vi "Config.vi"(8 "Error In":errorcluster) -> (0 "Error Out":errorcluster)   [LabVIEW 2019, in "Full User Interface.lvlib"]
uses:
  Full User Interface.lvlib
  <vilib>/Test Bench Framework/Test Executive.lvlibp/TestEngine/TestEngine/TestEngine/Typedefs/Local Report Configuration.ctl
  <vilib>/Test Bench Framework/Test Executive.lvlibp/TestEngine/TestEngine/TestEngine/Report Format.ctl
  <vilib>/Test Bench Framework/Test Executive.lvlibp/TestEngine/TestEngine/TestEngine/Typedefs/Database Configuration.ctl
  <vilib>/Test Bench Framework/Test Executive.lvlibp/TestEngine/TestEngine/TestEngine/Typedefs/TestEngine Cofiguration.ctl
  <vilib>/Test Bench Framework/Test Executive.lvlibp/TestEngine/TestEngine/TestEngine/Test Engine.lvclass
panel:
  in  "Cancel":bool
  in  "OK":bool
  in  "Tab Control":enum32{"Local Report", "Database", "Execute"}(tab)
  in  "Local Report Configuration":T1
  in  "Database Configuration":T3
  in  "Execute":T4
  # "*不合格时结束测试"
  # "*运行的时候忽略断点"
  # "*过滤测试项目，只显示有测试结果的测试项"
  # "*自动错误处理，测试项报错\n  时不显示弹窗"
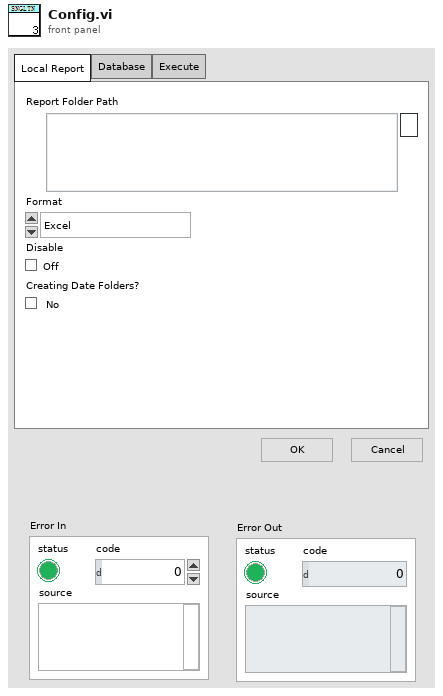
[diagram p1: front panel]
types:
  T1 = typedef "Test Executive.lvlibp/Test Engine.lvlib/Test Engine.lvclass/Local Report Configuration.ctl" = cluster{"Report Folder Path":path, "Format":T2, "Disable":bool, "Build Date Folder?":bool, "Execl Template Path":path}
  T2 = typedef "Test Executive.lvlibp/Test Engine.lvlib/Test Engine.lvclass/Report Format.ctl" = enum16{"Excel", "CSV(Tab)", "CSV(,)", "CSV(;)", "TEXT", "HTML"}
  T3 = typedef "Test Executive.lvlibp/Test Engine.lvlib/Test Engine.lvclass/Database Configuration.ctl" = cluster{"Connection String Expression":string, "Microsoft Data Link File":path, "Connection Type":enum16{"Use Connection String Expression", "Use Microsoft Data Link File"}, "Enable":bool}
  T4 = cluster{"Automatically handle TestVI error":cluster{"Enable":bool, "Handle":enum16{"Termination test", "Ignore error"}}, "Break on Failure":bool, "Ignore breakpoint":bool, "Filter Result":bool}
  T5 = enum32{"Invalid", "Standard", "Closed", "Hidden", "Minimized", "Maximized"}
  T6 = enum32{"invalid app kind", "Development System", "Run Time System", "Student Edition", "Embedded LabVIEW", "Evaluation", "Custom"}
  T7 = typedef "Test Executive.lvlibp/Test Engine.lvlib/Test Engine.lvclass/TestEngine Cofiguration.ctl" = cluster{"Break on Failure":bool, "Automatically handle TestVI error":cluster{"Enable":bool, "Handle":enum16{"Termination test", "Ignore error"}}, "Local Report Configuration":T1, "Database Configuration":T3, "Ignore breakpoint":bool, "Filter Result":bool}
  T8 = cluster{"Core":cluster{"Current VI Reference":refnum<vi>, "Close Panel on Exit?":bool}, "TestEngine Cofiguration":T7, "handle error":refnum<vi>, "Break on Failure":refnum<vi>, "Ignore breakpoint":refnum<vi>, "Filter Result":refnum<vi>, "Database Configuration":refnum<vi>, "Local Report Configuration":refnum<vi>, "Tab Control":refnum<vi>, "Execl Template Path":refnum<vi>}
  T9 = cluster{"Current VI Reference":refnum<vi>, "Close Panel on Exit?":bool}
  T10 = cluster{"Enable":bool, "Handle":enum16{"Termination test", "Ignore error"}}
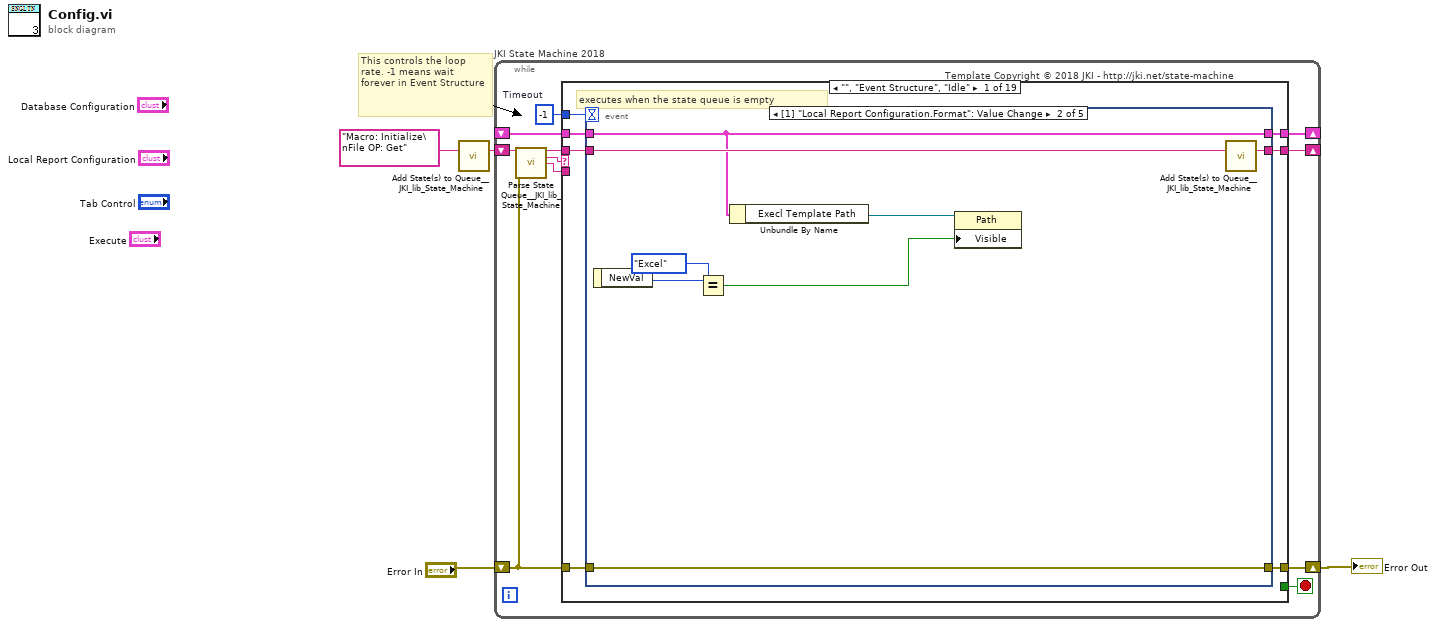
[diagram p0: block diagram]
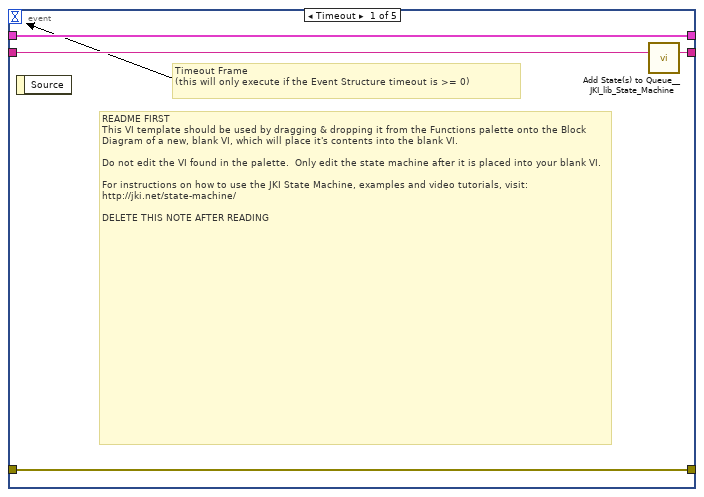
[diagram p2: hidden frame]
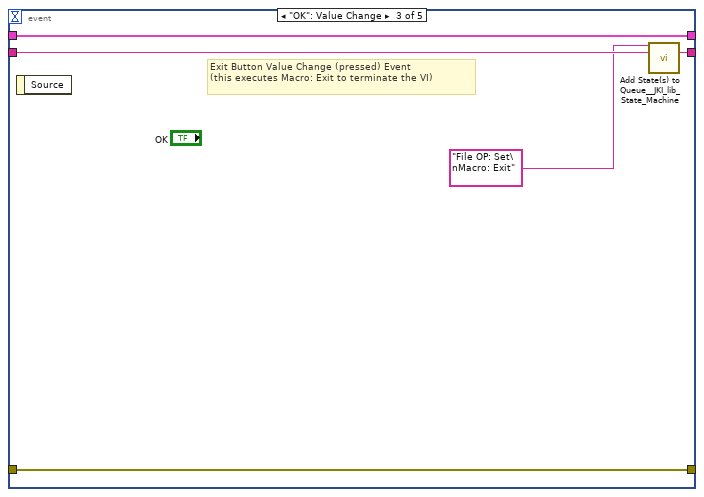
[diagram p3: hidden frame]
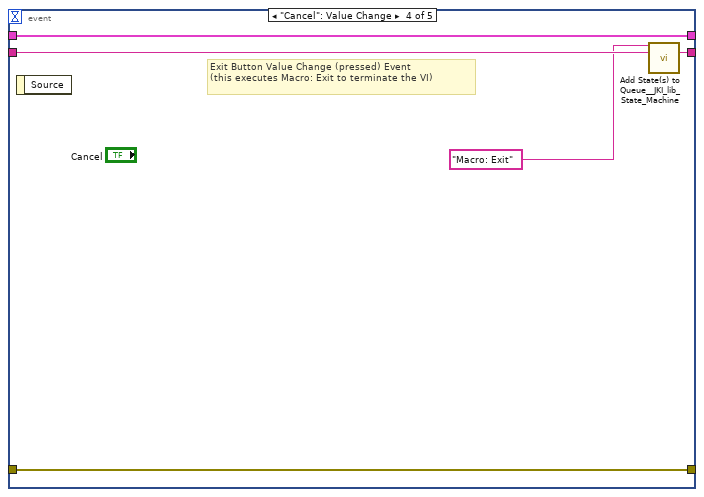
[diagram p4: hidden frame]
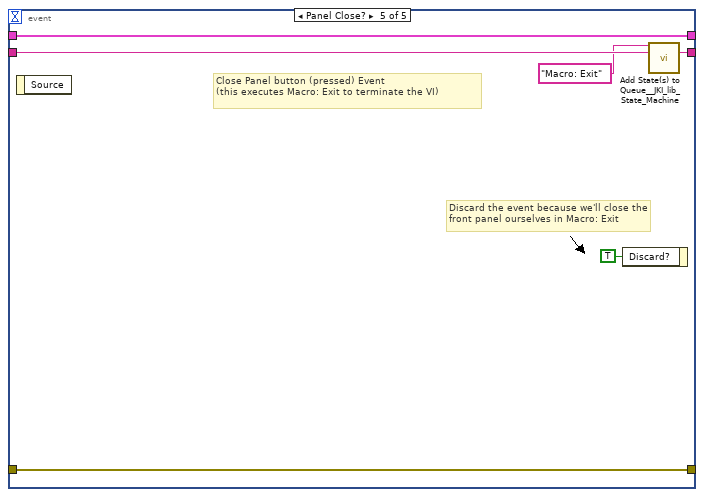
[diagram p5: hidden frame]
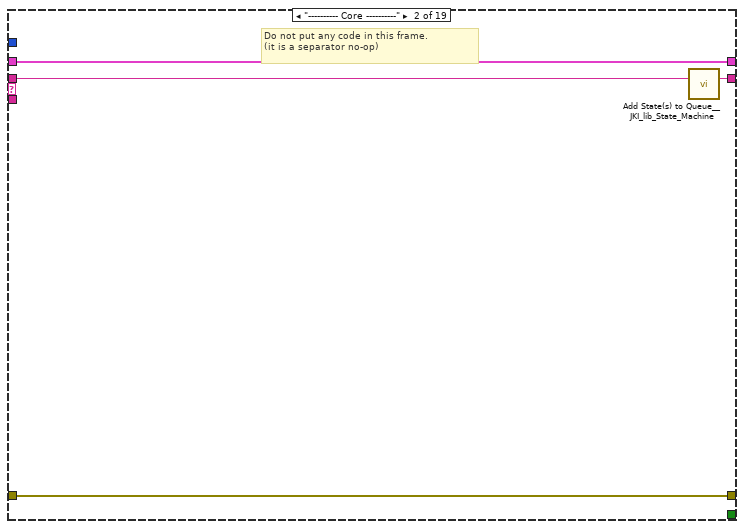
[diagram p6: hidden frame]
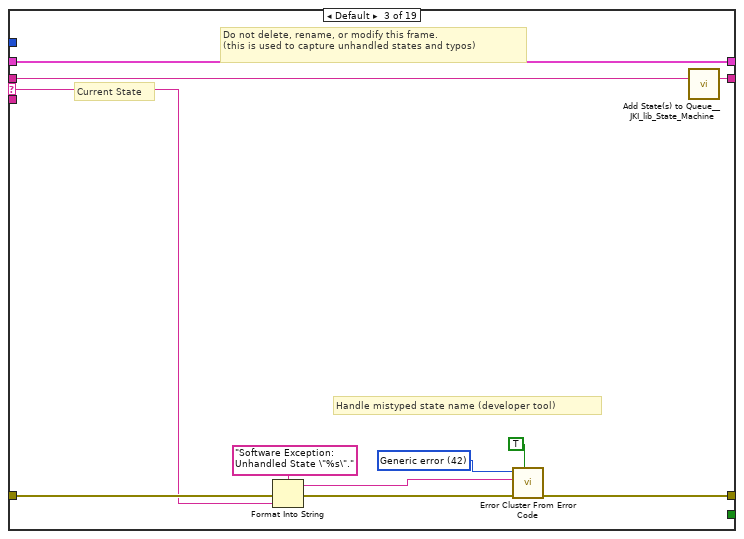
[diagram p7: hidden frame]
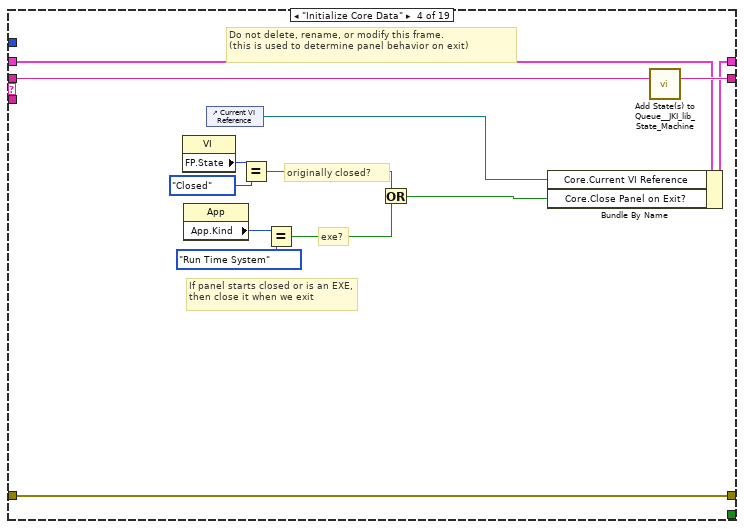
[diagram p8: hidden frame]
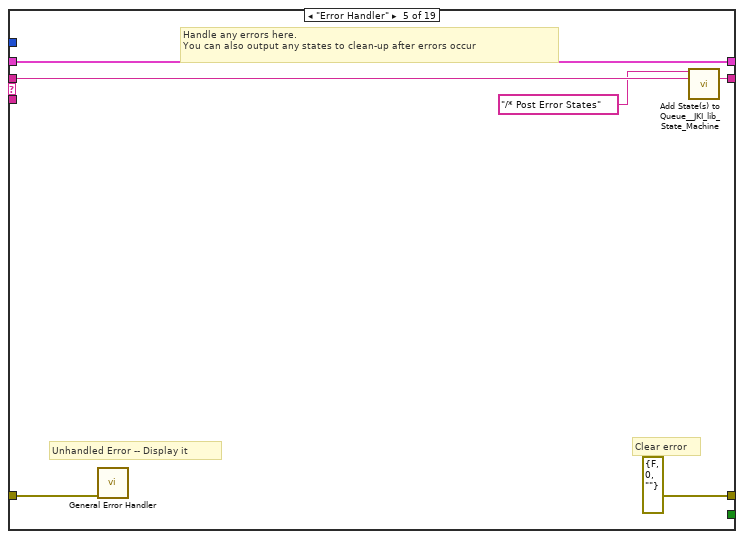
[diagram p9: hidden frame]
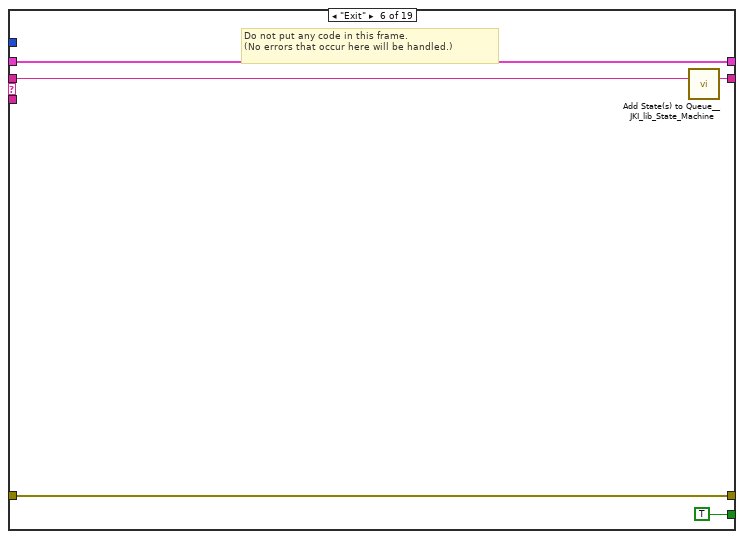
[diagram p10: hidden frame]
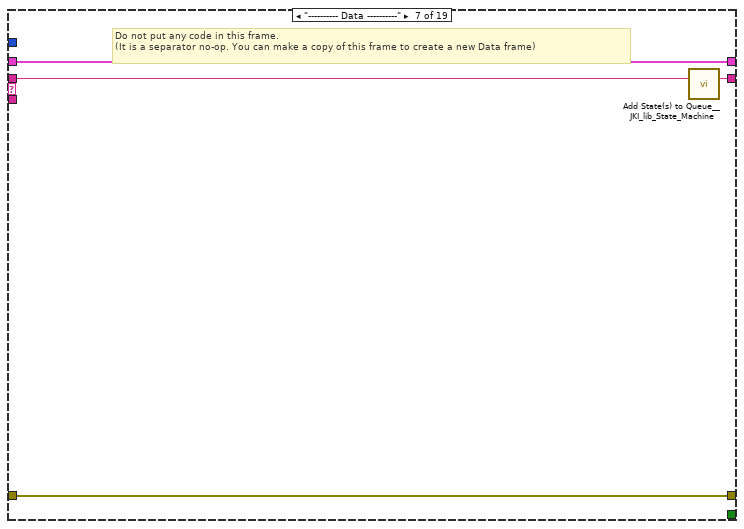
[diagram p11: hidden frame]
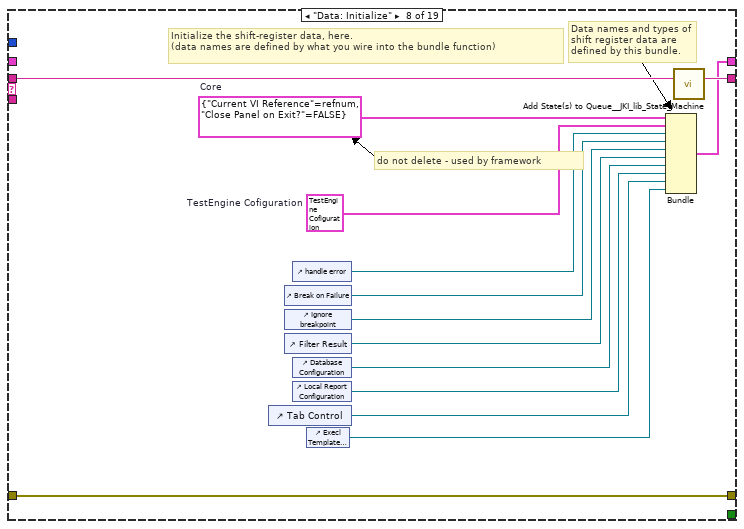
[diagram p12: hidden frame]
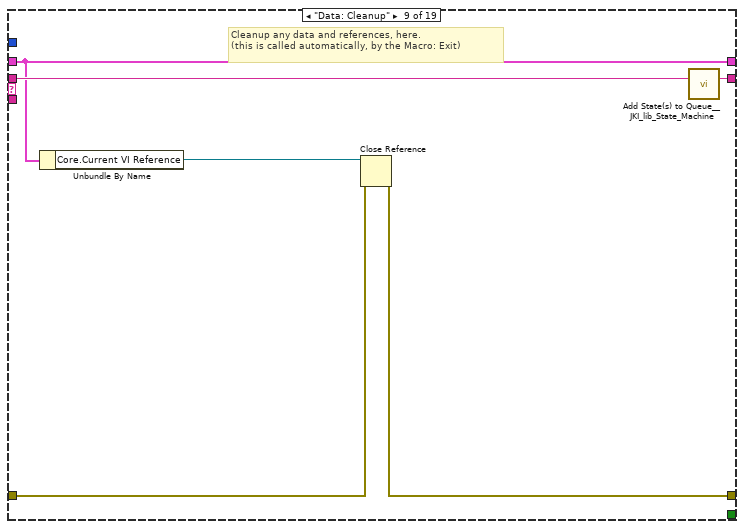
[diagram p13: hidden frame]
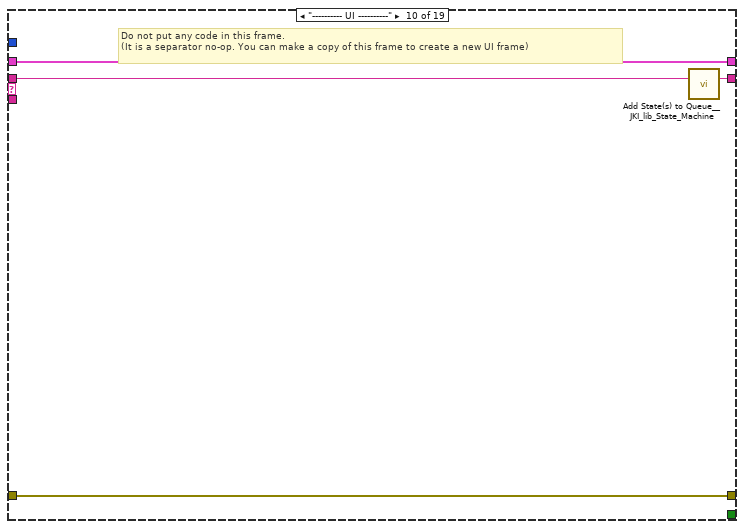
[diagram p14: hidden frame]
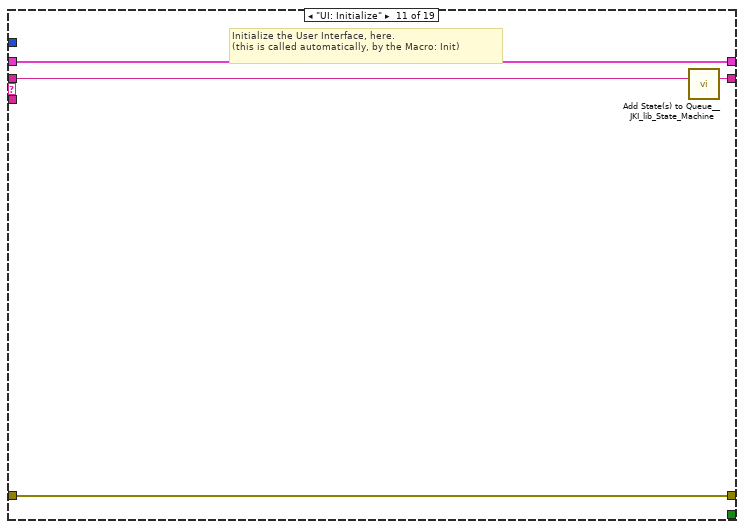
[diagram p15: hidden frame]
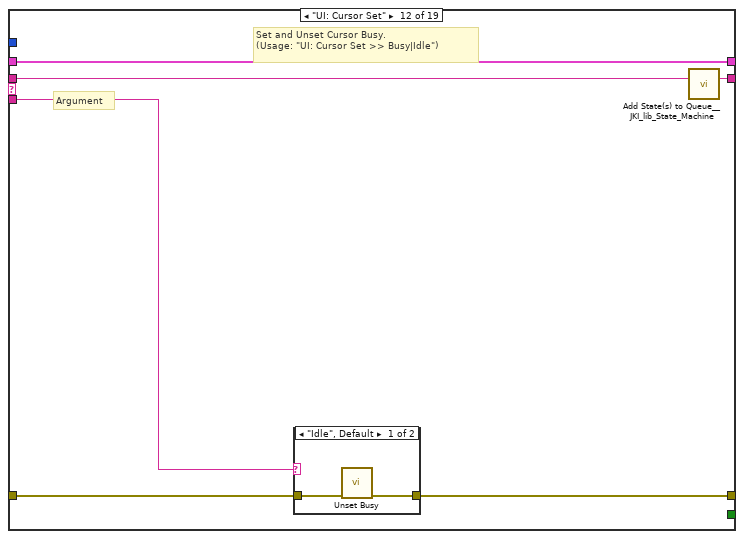
[diagram p16: hidden frame]
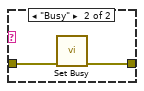
[diagram p17: hidden frame]
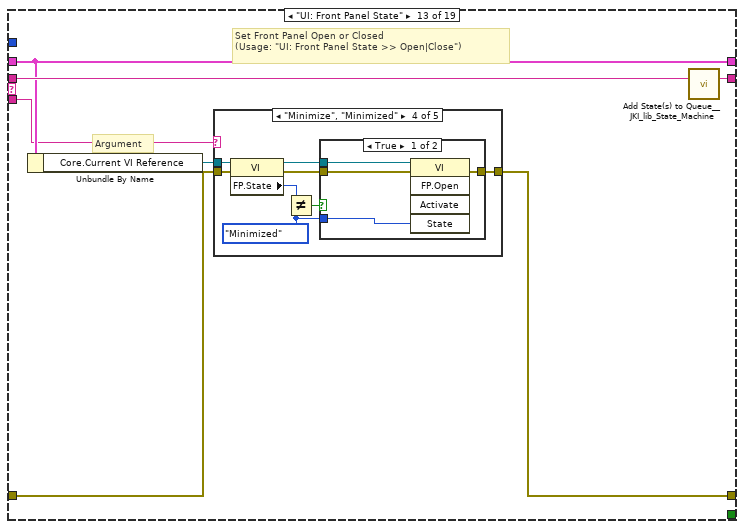
[diagram p18: hidden frame]
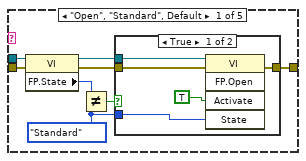
[diagram p19: hidden frame]
diagram:
  # "This controls the loop rate. -1 means wait forever in Event Structure"
  n1 = call <vilib>:"Add State(s) to Queue__JKI_lib_State_Machine.vi"("State(s) in (\"\")"="Macro: Initialize\nFile OP: Get") -> ("States Out"=w4:string)  [unwired: 14 in]
  n2 = while "JKI State Machine 2018" {
    shift-right: [w8] -> _
    shift-left: _ -> [w7]
    shift-right: [w11] -> w1
    shift-left: "Error In" -> [w5]
    shift-right: [w10] -> _
    shift-left: w4 -> [w12]
    stop <- w9 stop-if-true
    w6 = -1  # Timeout
    # "Template Copyright © 2018 JKI - http://jki.net/state-machine"
    n3 = call <vilib>:"Parse State Queue__JKI_lib_State_Machine.vi"("State Queue"=w12, "Error In (no error)"=w5) -> ("Remaining States"=w14:string, "Current State"=w15:string, "Arguments"=w13:string)  [unwired: 11 in]
    n4 = case shown="\"\", \"Event Structure\", \"Idle\"" w15 {
      selector: w15 -> [_ _ w55 _ _ _ _ _ _ _ _ _ _ _ _ _ _ _ _]
      tunnel: w14 -> [w22 w54 w59 w78 w84 w89 w93 w107 w113 w117 w121 w127 w138 w207 w212 w222 w226 w249 w269]
      tunnel: w13 -> [_ _ _ _ _ _ _ _ _ _ _ w122 w132 _ _ _ _ _ _]
      tunnel: w7 -> [w20 w51 w57 w71 w81 w87 w90 _ w108 w114 w119 w125 w134 w204 w209 w219 w223 w246 w260]
      tunnel: [w19 w52 w61 w75 errorcluster {"status"=FALSE, "code"=0, "source"=""} ("error out") w86 w91 w104 w109 w115 w118 w123 w135 w205 w210 w220 w224 w245 w252] -> w11
      tunnel: w5 -> [w18 w52 w60 w75 w80 w86 w91 w104 w110 w115 w118 w124 w136 w205 w210 w220 w224 w247 w267]
      tunnel: [w21 w53 w58 w77 w83 w88 w92 w106 w112 w116 w120 w126 w137 w206 w211 w221 w225 w248 w268] -> w10
      tunnel: [_ _ _ _ _ TRUE _ _ _ _ _ _ _ _ _ _ _ _ _] -> w9
      tunnel: [w17 w51 w57 w76 w81 w87 w90 w105 w108 w114 w119 w125 w134 w204 w209 w219 w223 w246 w260] -> w8
      tunnel: w6 -> [w16 _ _ _ _ _ _ _ _ _ _ _ _ _ _ _ _ _ _]
      frame "", "Event Structure", "Idle" {
        # "executes when the state queue is empty"
        n5 = event shown="[1] \"Local Report Configuration.Format\": Value Change" {
          selector: _ -> [_ _ _ _ _]
          dyn-events: _ -> [_ _ _ _ _]
          timeout: w16 -> [_ _ _ _ _]
          tunnel: w22 -> [w26 w34 w39 w44 w50]
          tunnel: [w25 w33 w38 w43 w49] -> w21
          tunnel: w20 -> [w23 w29 w36 w41 w47]
          tunnel: [w24 w32 w37 w42 w48] -> w19
          tunnel: w18 -> [w24 w32 w37 w42 w48]
          tunnel: [w23 w29 w36 w41 w47] -> w17
          event Timeout {
            # "README FIRST\nThis VI template should be used by dragging & dropping it from the Functions palette onto the Block Diagram of a new, blank VI, which will place it's contents into the blank VI.\n\nDo not edit the VI found in the palette.  Only edit the state machine after it is placed into your blank VI.\n\nFor instructions on how to use the JKI State Machine, examples and video tutorials, visit:\nhttp://jki.net/state-machine/\n\nDELETE THIS NOTE AFTER READING"
            # "Timeout Frame\n(this will only execute if the Event Structure timeout is >= 0)"
            n6 = event-data() -> ()  [unwired: 1 in, 1 out]
            n7 = call <vilib>:"Add State(s) to Queue__JKI_lib_State_Machine.vi"("State(s) in (\"\")"=w26) -> ("States Out"=w25:string)  [unwired: 14 in]
          }
          event Value Change {
            n8 = event-data() -> ("NewVal"=w31:T2)  [unwired: 1 in]
            n9 = Equal?(x=w31, y=Report_Format."Excel") -> (x = y?=w27:bool)
            n10 = Unbundle By Name(w29) -> ("Execl Template Path"=w28:refnum<vi>)
            n11 = property class="Path"(reference=w28, "Visible"=w27) -> ()  [unwired: 1 in, 2 out]
            n12 = call <vilib>:"Add State(s) to Queue__JKI_lib_State_Machine.vi"("State(s) in (\"\")"=w34) -> ("States Out"=w33:string)  [unwired: 14 in]
          }
          event "OK": Value Change {
            # "Exit Button Value Change (pressed) Event\n(this executes Macro: Exit to terminate the VI)"
            n13 = event-data() -> ()  [unwired: 1 in, 1 out]
            n14 = call <vilib>:"Add State(s) to Queue__JKI_lib_State_Machine.vi"("State(s) in Front (\"\")"="File OP: Set\nMacro: Exit", "State(s) in (\"\")"=w39) -> ("States Out"=w38:string)  [unwired: 13 in]
          }
          event "Cancel": Value Change {
            # "Exit Button Value Change (pressed) Event\n(this executes Macro: Exit to terminate the VI)"
            n15 = event-data() -> ()  [unwired: 1 in, 1 out]
            n16 = call <vilib>:"Add State(s) to Queue__JKI_lib_State_Machine.vi"("State(s) in Front (\"\")"="Macro: Exit", "State(s) in (\"\")"=w44) -> ("States Out"=w43:string)  [unwired: 13 in]
          }
          event Panel Close? {
            # "Discard the event because we'll close the front panel ourselves in Macro: Exit"
            # "Close Panel button (pressed) Event\n(this executes Macro: Exit to terminate the VI)"
            n17 = event-data() -> ()  [unwired: 1 in, 1 out]
            n18 = event-data("Discard?"=TRUE) -> ()  [unwired: 1 in, 1 out]
            n19 = call <vilib>:"Add State(s) to Queue__JKI_lib_State_Machine.vi"("State(s) in Front (\"\")"="Macro: Exit", "State(s) in (\"\")"=w50) -> ("States Out"=w49:string)  [unwired: 13 in]
          }
        }
      }
      frame "---------- Core ----------" {
        # "Do not put any code in this frame.\n(it is a separator no-op)"
        n20 = call <vilib>:"Add State(s) to Queue__JKI_lib_State_Machine.vi"("State(s) in (\"\")"=w54) -> ("States Out"=w53:string)  [unwired: 14 in]
      }
      frame Default {
        w64 = 42 items=["No error", "Argument error", "Memory is full", "Out of zone", "End of file", "File already open", "Generic file I/O error", "File not found", "File permission error", "Disk is full", "Duplicate path", "Too many files open", "System feature not enabled", "Resource file not found", "Cannot add resource", "Resource not found", "Image not found", "Image memory error", "Pen does not exist", "Config type invalid", "Config token not found", "Config parse error", "Config memory error", "Bad external code format", "Bad external code offset", "External code not present", "Null window", "Destroy window error", "Null menu", "Print aborted", "Bad print record", "Print driver error", "Windows error during printing", "Memory error during printing", "Print dialog error", "Generic print error", "Invalid device refnum", "Device not found", "Device parameter error", "Device unit error", "Cannot open device", "Device call aborted", "Generic error", "Cancelled by user", "Object ID too low", "Object ID too high", "Object not in heap", "Unknown heap", "Unknown object (invalid DefProc)", "Unknown object (DefProc not in table)", "Message out of range", "Invalid (null) method", "Unknown message", "Manager call not supported", "Bad address", "Network operation in progress", "Network operation timed out", "Connection is busy", "Network attribute not supported", "Network error", "Address in use", "System out of memory", "Connection aborted", "Connection refused", "Not connected", "Already connected", "Connection closed", "Initialization error (interapplication manager)", "Bad occurrence", "Wait on unbound occurrence handler", "Occurrence queue overflow", "Datalog type conflict", "Unused", "Unrecognized type (interapplication manager)", "Memory corrupt", "Failed to make temporary DLL", "Old CIN version", "Drag socket not found", "Failed to load drop-object", "Failed to register OLE object", "Failed to release OLE object", "Format specifier type mismatch", "Unknown format specifier", "Too few format specifiers", "Too many format specifiers", "Scan failed", "Newer CIN version", "Error converting to variant", "Runtime menu error", "Password tampered", "Variant attribute not found", "Incompatible variant data type", "Event data is not available", "Event Store is not present", "Occurrence is not found", "Event Queue is not created", "Event info is not available", "Refnum passed is NULL", "Error retrieving Class GUID", "Error retrieving CoClass GUID", "Error retrieving TypeLib GUID.", "Bad built application magic bytes.", "Specific driver is different from the specific driver associated with the Logical Name.", "There is no session opened to the class driver.", "Max Error", "MAX - Error with config objects", "MAX - Error loading configuration", "MAX - Group not supported"]
        # "Current State"
        # "Do not delete, rename, or modify this frame.\n(this is used to capture unhandled states and typos)"
        # "Handle mistyped state name (developer tool)"
        n21 = Format Into String(format string="Software Exception: Unhandled State \"%s\"." ("message"), error in=w60, w55) -> (resulting string=w63:string, error out=w62:errorcluster)  [unwired: 1 in]
        n22 = call <vilib>:"Error Cluster From Error Code.vi"("show call chain? (False)"=TRUE, "error in (no error)"=w62, "error message (\"\")"=w63, "error code (0)"=w64) -> ("error out"=w61:errorcluster)  [unwired: 5 in]
        n23 = call <vilib>:"Add State(s) to Queue__JKI_lib_State_Machine.vi"("State(s) in (\"\")"=w59) -> ("States Out"=w58:string)  [unwired: 14 in]
      }
      frame "Initialize Core Data" {
        # "Do not delete, rename, or modify this frame.\n(this is used to determine panel behavior on exit)"
        # "originally closed?"
        # "exe?"
        # "If panel starts closed or is an EXE, then close it when we exit"
        n24 = property class="VI"() -> ("FP.State"=w68:T5)  [unwired: 2 in, 2 out]
        n25 = property class="App"() -> ("App.Kind"=w74:T6)  [unwired: 2 in, 2 out]
        n26 = control-ref of="Current VI Reference"() -> (w69:refnum<vi>)
        n27 = Equal?(x=w68, y=T5."Closed" ("Front Panel Window:State")) -> (x = y?=w66:bool)
        n28 = Equal?(x=w74, y=T6."Run Time System" ("Application:Kind")) -> (x = y?=w72:bool)
        n29 = Or(x=w66, y=w72) -> (x .or. y?=w70:bool)
        n30 = Bundle By Name(cluster=w71, "Core.Current VI Reference"=w69, "Core.Close Panel on Exit?"=w70) -> (w76:T8)
        n31 = call <vilib>:"Add State(s) to Queue__JKI_lib_State_Machine.vi"("State(s) in (\"\")"=w78) -> ("States Out"=w77:string)  [unwired: 14 in]
      }
      frame "Error Handler" {
        # "Unhandled Error -- Display it"
        # "Handle any errors here.\nYou can also output any states to clean-up after errors occur"
        # "Clear error"
        n32 = call <vilib>:"General Error Handler.vi"("error in (no error)"=w80) -> ()  [unwired: 10 in, 5 out]
        n33 = call <vilib>:"Add State(s) to Queue__JKI_lib_State_Machine.vi"("State(s) in Front (\"\")"="/* Post Error States", "State(s) in (\"\")"=w84) -> ("States Out"=w83:string)  [unwired: 13 in]
      }
      frame "Exit" {
        # "Do not put any code in this frame.\n(No errors that occur here will be handled.)"
        n34 = call <vilib>:"Add State(s) to Queue__JKI_lib_State_Machine.vi"("State(s) in (\"\")"=w89) -> ("States Out"=w88:string)  [unwired: 14 in]
      }
      frame "---------- Data ----------" {
        # "Do not put any code in this frame.\n(It is a separator no-op. You can make a copy of this frame to create a new Data frame)"
        n35 = call <vilib>:"Add State(s) to Queue__JKI_lib_State_Machine.vi"("State(s) in (\"\")"=w93) -> ("States Out"=w92:string)  [unwired: 14 in]
      }
      frame "Data: Initialize" {
        w102 = T7 {"Break on Failure"=FALSE, "Automatically handle TestVI error"={"Enable"=FALSE, "Handle"=enum."Termination test"}, "Local Report Configuration"={"Report Folder Path"=path "", "Format"=enum."Excel", "Disable"=FALSE, "Build Date Folder?"=FALSE, "Execl Template Path"=path ""}, "Database Configuration"={"Connection String Expression"="", "Microsoft Data Link File"=path "", "Connection Type"=enum."Use Connection String Expression", "Enable"=FALSE}, "Ignore breakpoint"=FALSE, "Filter Result"=FALSE}  # TestEngine Cofiguration
        w103 = T9 {"Current VI Reference"=refnum, "Close Panel on Exit?"=FALSE}  # Core
        # "do not delete - used by framework"
        # "Data names and types of shift register data are defined by this bundle."
        # "Initialize the shift-register data, here.\n(data names are defined by what you wire into the bundle function)"
        n36 = control-ref of="Tab Control"() -> (w95:refnum<vi>)
        n37 = control-ref of="Break on Failure"() -> (w100:refnum<vi>)
        n38 = control-ref of="Ignore breakpoint"() -> (w99:refnum<vi>)
        n39 = control-ref of="Filter Result"() -> (w98:refnum<vi>)
        n40 = control-ref of="handle error"() -> (w101:refnum<vi>)
        n41 = control-ref of="Database Configuration"() -> (w97:refnum<vi>)
        n42 = control-ref of="Local Report Configuration"() -> (w96:refnum<vi>)
        n43 = control-ref of="Execl Template Path"() -> (w94:refnum<vi>)
        n44 = Bundle("Core"=w103, "TestEngine Cofiguration"=w102, "handle error"=w101, "Break on Failure"=w100, "Ignore breakpoint"=w99, "Filter Result"=w98, "Database Configuration"=w97, "Local Report Configuration"=w96, "Tab Control"=w95, "Execl Template Path"=w94) -> (w105:T8)  [unwired: 1 in]
        n45 = call <vilib>:"Add State(s) to Queue__JKI_lib_State_Machine.vi"("State(s) in (\"\")"=w107) -> ("States Out"=w106:string)  [unwired: 14 in]
      }
      frame "Data: Cleanup" {
        # "Cleanup any data and references, here.\n(this is called automatically, by the Macro: Exit)"
        n46 = Unbundle By Name(w108) -> ("Core.Current VI Reference"=w111:refnum<vi>)
        n47 = Close Reference(reference=w111, error in (no error)=w110) -> (error out=w109:errorcluster)
        n48 = call <vilib>:"Add State(s) to Queue__JKI_lib_State_Machine.vi"("State(s) in (\"\")"=w113) -> ("States Out"=w112:string)  [unwired: 14 in]
      }
      frame "---------- UI ----------" {
        # "Do not put any code in this frame.\n(It is a separator no-op. You can make a copy of this frame to create a new UI frame)"
        n49 = call <vilib>:"Add State(s) to Queue__JKI_lib_State_Machine.vi"("State(s) in (\"\")"=w117) -> ("States Out"=w116:string)  [unwired: 14 in]
      }
      frame "UI: Initialize" {
        # "Initialize the User Interface, here.\n(this is called automatically, by the Macro: Init)"
        n50 = call <vilib>:"Add State(s) to Queue__JKI_lib_State_Machine.vi"("State(s) in (\"\")"=w121) -> ("States Out"=w120:string)  [unwired: 14 in]
      }
      frame "UI: Cursor Set" {
        # "Argument"
        # "Set and Unset Cursor Busy.\n(Usage: \"UI: Cursor Set >> Busy|Idle\")"
        n51 = case shown="\"Idle\", Default" w122 {
          tunnel: w124 -> [w129 w131]
          tunnel: [w128 w130] -> w123
          frame "Idle", Default {
            n52 = call <vilib>:"Unset Busy.vi"("error in (no error)"=w129) -> ("error out"=w128:errorcluster)  [unwired: 10 in]
          }
          frame "Busy" {
            n53 = call <vilib>:"Set Busy.vi"("error in (no error)"=w131) -> ("error out"=w130:errorcluster)  [unwired: 9 in, 1 out]
          }
        }
        n54 = call <vilib>:"Add State(s) to Queue__JKI_lib_State_Machine.vi"("State(s) in (\"\")"=w127) -> ("States Out"=w126:string)  [unwired: 14 in]
      }
      frame "UI: Front Panel State" {
        # "Argument"
        # "Set Front Panel Open or Closed\n(Usage: \"UI: Front Panel State >> Open|Close\")"
        n55 = Unbundle By Name(w134) -> ("Core.Current VI Reference"=w133:refnum<vi>)
        n56 = case shown="\"Minimize\", \"Minimized\"" w132 {
          tunnel: w136 -> [w144 w159 w170 w183 w196]
          tunnel: [w146 w160 w172 w185 w198] -> w135
          tunnel: w133 -> [w145 w157 w171 w184 w197]
          frame "Open", "Standard", Default {
            w139 = T5."Standard" ("State")
            n57 = property class="VI"(reference=w145, error in=w144) -> (reference out=w142:refnum<vi>, error out=w143:errorcluster, "FP.State"=w141:T5)
            n58 = Not Equal?(x=w141, y=w139) -> (x != y?=w140:bool)
            n59 = case shown="True" w140 {
              tunnel: [w150 w152] -> w146
              tunnel: w143 -> [w149 w152]
              tunnel: w142 -> [w148 _]
              tunnel: w139 -> [w147 _]
              frame True {
                n60 = invoke class="VI" method="FP.Open"(reference=w148, error in=w149, "Activate"=TRUE, "State"=w147) -> (error out=w150:errorcluster)  [unwired: 1 in, 4 out]
              }
              frame False {
              }
            }
          }
          frame "Close", "Closed" {
            n61 = property class="VI"(reference=w157, error in=w159) -> (reference out=w156:refnum<vi>, error out=w158:errorcluster, "FP.State"=w154:T5)
            n62 = Not Equal?(x=w154, y=T5."Closed" ("Front Panel Window:State")) -> (x != y?=w153:bool)
            n63 = case shown="True" w153 {
              tunnel: [w161 w164] -> w160
              tunnel: w158 -> [w161 w163]
              tunnel: w156 -> [_ w162]
              frame False {
              }
              frame True {
                n64 = invoke class="VI" method="FP.Close"(reference=w162, error in=w163) -> (error out=w164:errorcluster)  [unwired: 1 in, 2 out]
              }
            }
          }
          frame "Hidden", "Hide" {
            w165 = T5."Hidden" ("State")
            n65 = property class="VI"(reference=w171, error in=w170) -> (reference out=w168:refnum<vi>, error out=w169:errorcluster, "FP.State"=w167:T5)
            n66 = Not Equal?(x=w167, y=w165) -> (x != y?=w166:bool)
            n67 = case shown="True" w166 {
              tunnel: [w176 w177] -> w172
              tunnel: w169 -> [w175 w177]
              tunnel: w168 -> [w174 _]
              tunnel: w165 -> [w173 _]
              frame True {
                n68 = invoke class="VI" method="FP.Open"(reference=w174, error in=w175, "State"=w173) -> (error out=w176:errorcluster)  [unwired: 2 in, 4 out]
              }
              frame False {
              }
            }
          }
          frame "Minimize", "Minimized" {
            w178 = T5."Minimized" ("State")
            n69 = property class="VI"(reference=w184, error in=w183) -> (reference out=w181:refnum<vi>, error out=w182:errorcluster, "FP.State"=w180:T5)
            n70 = Not Equal?(x=w180, y=w178) -> (x != y?=w179:bool)
            n71 = case shown="True" w179 {
              tunnel: [w189 w190] -> w185
              tunnel: w182 -> [w188 w190]
              tunnel: w181 -> [w187 _]
              tunnel: w178 -> [w186 _]
              frame True {
                n72 = invoke class="VI" method="FP.Open"(reference=w187, error in=w188, "State"=w186) -> (error out=w189:errorcluster)  [unwired: 2 in, 4 out]
              }
              frame False {
              }
            }
          }
          frame "Maximize", "Maximized" {
            w191 = T5."Maximized" ("State")
            n73 = property class="VI"(reference=w197, error in=w196) -> (reference out=w194:refnum<vi>, error out=w195:errorcluster, "FP.State"=w193:T5)
            n74 = Not Equal?(x=w193, y=w191) -> (x != y?=w192:bool)
            n75 = case shown="True" w192 {
              tunnel: [w202 w203] -> w198
              tunnel: w195 -> [w201 w203]
              tunnel: w194 -> [w200 _]
              tunnel: w191 -> [w199 _]
              frame True {
                n76 = invoke class="VI" method="FP.Open"(reference=w200, error in=w201, "State"=w199) -> (error out=w202:errorcluster)  [unwired: 2 in, 4 out]
              }
              frame False {
              }
            }
          }
        }
        n77 = call <vilib>:"Add State(s) to Queue__JKI_lib_State_Machine.vi"("State(s) in (\"\")"=w138) -> ("States Out"=w137:string)  [unwired: 14 in]
      }
      frame "---------- Macro ----------" {
        # "Do not put any code in this frame.\n(It is a separator no-op. You can make a copy of this frame to create a new Macro frame)"
        n78 = call <vilib>:"Add State(s) to Queue__JKI_lib_State_Machine.vi"("State(s) in (\"\")"=w207) -> ("States Out"=w206:string)  [unwired: 14 in]
      }
      frame "Macro: Initialize" {
        w208 = "Data: Initialize\nInitialize Core Data\nUI: Initialize\nUI: Front Panel State >> Open"  # Data: Initialize Initialize Core Data UI: Initialize UI: Front Panel State >> Open
        # "Initialization Macro\n(This is called once, when the VI starts)"
        n79 = call <vilib>:"Add State(s) to Queue__JKI_lib_State_Machine.vi"("State(s) in Front (\"\")"=w208, "State(s) in (\"\")"=w212) -> ("States Out"=w211:string)  [unwired: 13 in]
      }
      frame "Macro: Exit" {
        # "Exit Macro\n(This is called once, when the VI exits)"
        n80 = Unbundle By Name(w219) -> ("Core.Close Panel on Exit?"=w218:bool)
        n81 = Select(t="UI: Front Panel State >> Close", s=w218, f="") -> (s? t:f=w215:string)
        n82 = call <vilib>:"Add State(s) to Queue__JKI_lib_State_Machine.vi"("State(s) in (\"\")"=w215, "State(s) at Back (\"\")"="Data: Cleanup\nExit") -> ("States Out"=w213:string)  [unwired: 13 in]
        n83 = call <vilib>:"Add State(s) to Queue__JKI_lib_State_Machine.vi"("State(s) in Front (\"\")"=w213, "State(s) in (\"\")"=w222) -> ("States Out"=w221:string)  [unwired: 13 in]
      }
      frame "---------- File OP ----------" {
        # "Your code here.\n(You can make a copy of, or modify, this frame)"
        n84 = call <vilib>:"Add State(s) to Queue__JKI_lib_State_Machine.vi"("State(s) in (\"\")"=w226) -> ("States Out"=w225:string)  [unwired: 14 in]
      }
      frame "File OP: Get" {
        # "Your code here.\n(You can make a copy of, or modify, this frame)"
        n85 = call "Get Config.vi"() -> ("error out"=w244:errorcluster, "Configur"=w243:T7)  [unwired: 10 in]
        n86 = Unbundle By Name(w246) -> ("Execl Template Path"=w232:refnum<vi>, "Break on Failure"=w242:refnum<vi>, "handle error"=w240:refnum<vi>, "Local Report Configuration"=w239:refnum<vi>, "Database Configuration"=w238:refnum<vi>, "Ignore breakpoint"=w236:refnum<vi>, "Filter Result"=w234:refnum<vi>)
        n87 = Unbundle(w243) -> ("Break on Failure"=w241:bool, "Automatically handle TestVI error"=w231:T10, "Local Report Configuration"=w230:T1, "Database Configuration"=w237:T3, "Ignore breakpoint"=w235:bool, "Filter Result"=w233:bool)
        n88 = property class="Bool (strict)"(reference=w234, "Value"=w233) -> ()  [unwired: 1 in, 2 out]
        n89 = property class="Bool (strict)"(reference=w236, "Value"=w235) -> ()  [unwired: 1 in, 2 out]
        n90 = property class="Clust (strict)"(reference=w238, "Value"=w237) -> ()  [unwired: 1 in, 2 out]
        n91 = property class="Clust (strict)"(reference=w239, "Value"=w230) -> ()  [unwired: 1 in, 2 out]
        n92 = Merge Errors(w244, w247) -> (w245:errorcluster)
        n93 = Unbundle By Name(w230) -> ("Format"=w229:T2)
        n94 = property class="Clust (strict)"(reference=w240, "Value"=w231) -> ()  [unwired: 1 in, 2 out]
        n95 = Equal?(x=w229, y=Report_Format."Excel") -> (x = y?=w227:bool)
        n96 = property class="Bool (strict)"(reference=w242, "Value"=w241) -> ()  [unwired: 1 in, 2 out]
        n97 = property class="Path"(reference=w232, "Visible"=w227) -> ()  [unwired: 1 in, 2 out]
        n98 = call <vilib>:"Add State(s) to Queue__JKI_lib_State_Machine.vi"("State(s) in (\"\")"=w249) -> ("States Out"=w248:string)  [unwired: 14 in]
      }
      frame "File OP: Set" {
        w250 = T7 {"Break on Failure"=FALSE, "Automatically handle TestVI error"={"Enable"=FALSE, "Handle"=enum."Termination test"}, "Local Report Configuration"={"Report Folder Path"=path "", "Format"=enum."Excel", "Disable"=FALSE, "Build Date Folder?"=FALSE, "Execl Template Path"=path ""}, "Database Configuration"={"Connection String Expression"="", "Microsoft Data Link File"=path "", "Connection Type"=enum."Use Connection String Expression", "Enable"=FALSE}, "Ignore breakpoint"=FALSE, "Filter Result"=FALSE}  # Configur
        # "Template Separator\n(You can make a copy of, or modify, this frame)"
        n99 = Unbundle By Name(w260) -> ("Break on Failure"=w266:refnum<vi>, "handle error"=w265:refnum<vi>, "Local Report Configuration"=w264:refnum<vi>, "Database Configuration"=w263:refnum<vi>, "Ignore breakpoint"=w262:refnum<vi>, "Filter Result"=w261:refnum<vi>)
        n100 = property class="Bool (strict)"(reference=w261) -> ("Value"=w254:bool)  [unwired: 1 in, 2 out]
        n101 = property class="Bool (strict)"(reference=w262) -> ("Value"=w255:bool)  [unwired: 1 in, 2 out]
        n102 = property class="Clust (strict)"(reference=w263) -> ("Value"=w256:T3)  [unwired: 1 in, 2 out]
        n103 = property class="Clust (strict)"(reference=w264) -> ("Value"=w257:T1)  [unwired: 1 in, 2 out]
        n104 = property class="Clust (strict)"(reference=w265) -> ("Value"=w258:T10)  [unwired: 1 in, 2 out]
        n105 = property class="Bool (strict)"(reference=w266) -> ("Value"=w259:bool)  [unwired: 1 in, 2 out]
        n106 = Bundle(cluster=w250, "Break on Failure"=w259, "Automatically handle TestVI error"=w258, "Local Report Configuration"=w257, "Database Configuration"=w256, "Ignore breakpoint"=w255, "Filter Result"=w254) -> (w253:T7)
        n107 = call "Set Config.vi"("Configur"=w253) -> ("error out"=w251:errorcluster)  [unwired: 10 in]
        n108 = call <vilib>:"Add State(s) to Queue__JKI_lib_State_Machine.vi"("State(s) in (\"\")"=w269) -> ("States Out"=w268:string)  [unwired: 14 in]
        n109 = Merge Errors(w251, w267) -> (w252:errorcluster)
      }
    }
  }
  "Error Out" <- w1
